vi "Load App.vi"(8 "Error In":errorcluster, 9 "Open Actor Core front panel? (F)":bool, 10 "Application Controller.lvclass":refnum<class "Application Controller.lvclass">, 11 "Status Notifier":refnum<notifier>) -> (0 "Error Out":errorcluster)   [LabVIEW 2016, in "Application Controller.lvclass"]
uses:
  Application Controller.lvclass
  C:/github/LabActor/Template Module/Template Module.lvclass
  C:/Program Files (x86)/National Instruments/LabVIEW 2016/vi.lib/ActorFramework/Actor/Actor.lvclass
  Template Module/Template Module.lvclass/Template Module.ctl
  Application Controller.lvclass/Application Controller.ctl
  Template Module/Write Name.vi
  Write Launch Notifier.vi
  Write Start-up configuration file.vi
  <vilib>/ActorFramework/Actor/Actor.lvclass
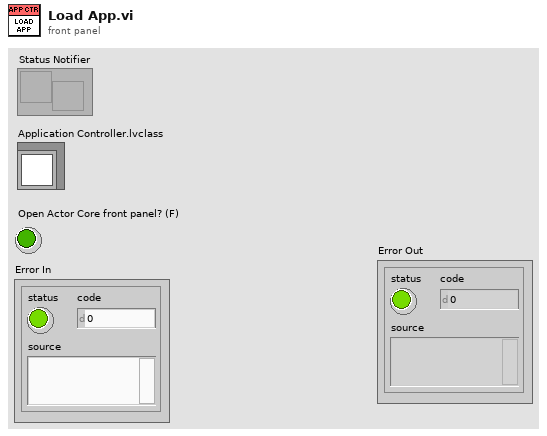
[diagram p1: front panel]
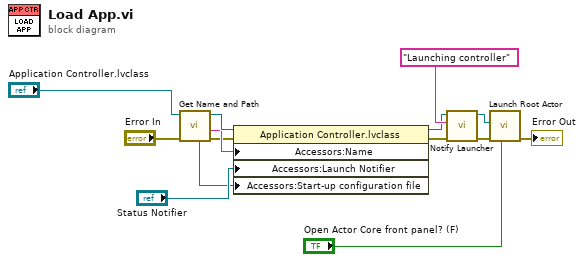
[diagram p0: block diagram]
diagram:
  n1 = call-dynamic "Get Name and Path.vi"("error in (no error)"="Error In", "Application Controller in"="Application Controller.lvclass") -> ("error out"=w3:errorcluster, "Name"=w4:string, "Application Controller out"=w5:refnum<class "Application Controller.lvclass">, "Start-up configuration path"=w1:path)  [unwired: 5 in, 1 out]
  n2 = property class="Application Controller.lvclass"(reference=w5, error in=w3, "Accessors:Name"=w4, "Accessors:Launch Notifier"="Status Notifier", "Accessors:Start-up configuration file"=w1) -> (reference out=w7:refnum<class "Application Controller.lvclass">, error out=w9:errorcluster)
  n3 = call-dynamic "Notify Launcher.vi"("error in (no error)"=w9, "Notification"="Launching controller" ("notification"), "Application Controller in"=w7) -> ("error out"=w12:errorcluster, "Application Controller out"=w13:refnum<class "Application Controller.lvclass">)  [unwired: 7 in]
  n4 = call <vilib>:"Launch Root Actor.vi"("Open Actor Core front panel? (F)"="Open Actor Core front panel? (F)", "error in (no error)"=w12, "Actor"=w13) -> ("error out"=→"Error Out":errorcluster)  [unwired: 7 in, 1 out]
